vi "Resize UI.vi"(11 "UI Refs In":T1) -> (2 "Page Size":dbl, 3 "UI Refs":T1)   [LabVIEW 2020, in "OOPanel.lvlib" / "ArrayManager.lvclass"]
uses:
  ArrayManager.lvclass
  UI Refs.ctl
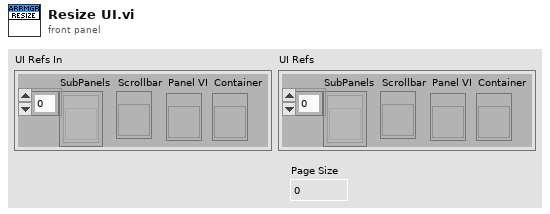
[diagram p1: front panel]
types:
  T1 = typedef "OOPanel.lvlib/ArrayManager.lvclass/UI Refs.ctl" = cluster{"SubPanels":refnum<vi>[], "Scrollbar":refnum<vi>, "Panel VI":refnum<vi>, "Container":refnum<vi>}
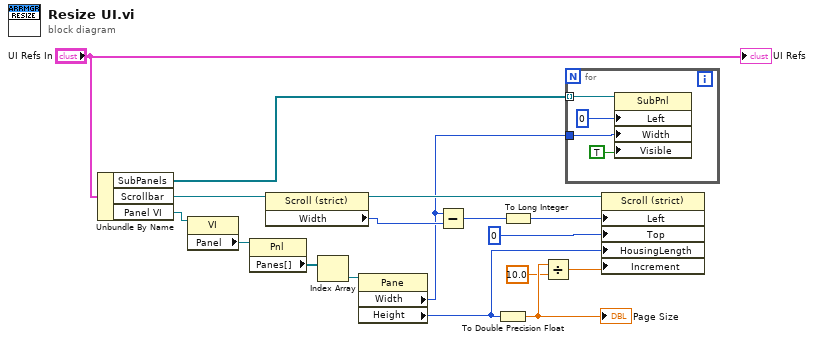
[diagram p0: block diagram]
diagram:
  n1 = Unbundle By Name("UI Refs In") -> ("SubPanels"=w9:refnum<vi>[], "Scrollbar"=w15:refnum<vi>, "Panel VI"=w7:refnum<vi>)
  n2 = property class="VI"(reference=w7) -> ("Panel"=w17:refnum<vi>)  [unwired: 1 in, 2 out]
  n3 = property class="Pnl"(reference=w17) -> ("Panes[]"=w11:refnum<vi>[])  [unwired: 1 in, 2 out]
  n4 = property class="Scroll (strict)"(reference=w15) -> (reference out=w14:refnum<vi>, "Width"=w2:u32)  [unwired: 1 in, 1 out]
  n5 = Index Array(array=w11) -> (element=w10:refnum<vi>)  [unwired: 1 in]
  n6 = property class="Pane"(reference=w10) -> ("Width"=w1:u32, "Height"=w6:u32)  [unwired: 1 in, 2 out]
  n7 = Subtract(x=w1, y=w2) -> (x-y=w8:u32)
  n8 = To Double Precision Float(number=w6) -> (double precision float=w5:dbl)
  "Page Size" <- w5
  n9 = To Long Integer(number=w8) -> (32bit integer=w13:i32)
  n10 = Divide(x=w5, y=10.0) -> (x/y=w3:dbl)
  n11 = for {
    tunnel: w9 -> [w21] mode=indexing
    tunnel: w1 -> [w19]
    n12 = property class="SubPnl"(reference=w21, "Left"=0 ("Position:Left"), "Width"=w19, "Visible"=TRUE) -> ()  [unwired: 1 in, 2 out]
  }
  n13 = property class="Scroll (strict)"(reference=w14, "Left"=w13, "Top"=0 ("Position:Top"), "HousingLength"=w6, "Increment"=w3) -> ()  [unwired: 1 in, 2 out]
  "UI Refs" <- "UI Refs In"
